vi "writeDO.vi"(8 "error in":errorcluster, 10 "Digital Signal Level":T1, 11 "DAQmx Global Channel":refnum<k21>) -> (0 "error out":errorcluster)   [LabVIEW 2015]
uses:
  Typedefs/Digital Signal Level.ctl
  <vilib>/DAQmx/write.llb/DAQmx Write (Digital Bool 1Line 1Point).vi
  <vilib>/DAQmx/miscellaneous.llb/DAQmx Fill In Error Info.vi
  Typedefs/ILCBTTypedefs.lvlib
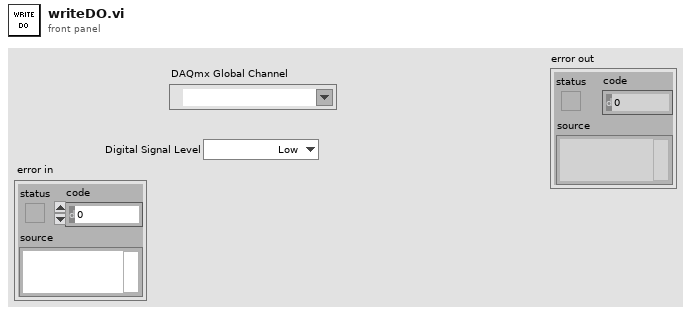
[diagram p1: front panel]
types:
  T1 = typedef "ILCBTTypedefs.lvlib/Digital Signal Level.ctl" = enum16{"Low", "High"}
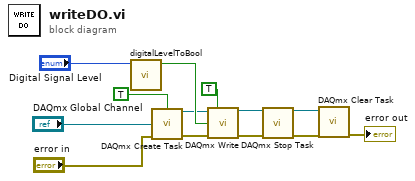
[diagram p0: block diagram]
diagram:
  n1 = call "digitalLevelToBool.vi"("Digital Signal Level"="Digital Signal Level") -> ("Bool?"=w7:bool)  [unwired: 10 in]
  n2 = call <vilib>:"DAQmx Create Task.vi"("auto cleanup"=TRUE, "global virtual channels"="DAQmx Global Channel", "error in"="error in") -> ("task out"=w2:refnum<k21>, "error out"=w1:errorcluster)  [unwired: 11 in]
  n3 = call-poly <vilib>:"DAQmx Write.vi"("task/channels in"=w2, "auto start"=TRUE, "data"=w7, "error in"=w1) -> ("task out"=w4:refnum<k21>, "error out"=w3:errorcluster)  [unwired: 9 in, 1 out]
  n4 = call <vilib>:"DAQmx Stop Task.vi"("task/channels in"=w4, "error in"=w3) -> ("task out"=w13:refnum<k21>, "error out"=w12:errorcluster)  [unwired: 12 in]
  n5 = call <vilib>:"DAQmx Clear Task.vi"("task in"=w13, "error in"=w12) -> ("error out"=→"error out":errorcluster)  [unwired: 13 in]
